vi "Advanced Buffer Configuration.vi"(0 "VISA resource name":refnum<visa-resource-name>, 1 "Enable Buffer Cache Mode (Disable)":bool, 5 "Buffer Name":string, 7 "Buffer Fill Mode (Fill_Once)":enum16{"FILL_ONCE", "FILL_WINDOW"}(ring), 9 "Buffer Fillcount":u16, 11 "error in (no error)":errorcluster) -> (4 "VISA resource name out":refnum<visa-resource-name>, 15 "error out":errorcluster)   [LabVIEW 2009, in "Keithley 2600 Series.lvlib"]
doc: "This VI allows advanced control over buffer features such as enabling cache mode, cache mode behavior and how many reading should be cached.\n\n<b>Functions and Attributes Used</b>\nbuffer.cachemode\nbuffer.fillmode\nbuffer.fillcount"
uses:
  <instrlib>/Keithley 2600 Series/Keithley 2600 Series.lvlib
  <instrlib>/Keithley 2600 Series/Private/GlobalVariables.vi
panel:
  # "(c) 2010 Keithley Instruments, Inc.  ALL RIGHTS RESERVED."
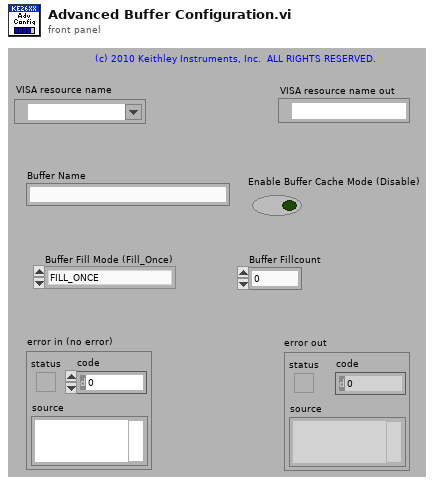
[diagram p1: front panel]
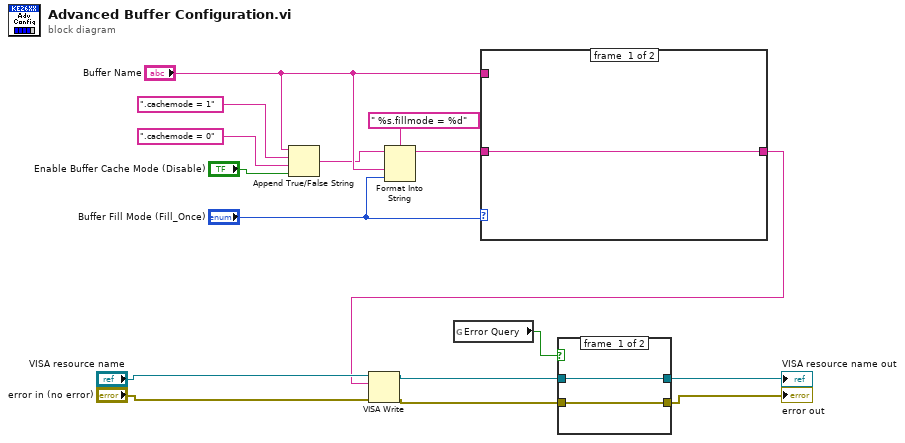
[diagram p0: block diagram]
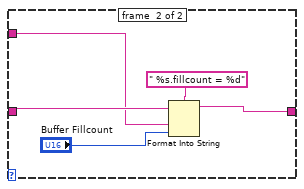
[diagram p2: hidden frame]
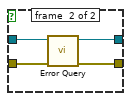
[diagram p3: hidden frame]
diagram:
  n1 = Append True/False String(1:"Enable Buffer Cache Mode (Disable)", 2:".cachemode = 0", 3:".cachemode = 1", 4:"Buffer Name") -> (0:w1:string)
  n2 = Format Into String(format string=" %s.fillmode = %d", initial string=w1, "Buffer Name", "Buffer Fill Mode (Fill_Once)") -> (resulting string=w4:string)  [unwired: 1 in, 1 out]
  n3 = global read "GlobalVariables.vi" "Error Query"() -> (w16:bool)
  n4 = case shown="\"FILL_ONCE\", Default" "Buffer Fill Mode (Fill_Once)" {
    tunnel: w4 -> [w17 w22]
    tunnel: "Buffer Name" -> [_ w21]
    tunnel: [w17 w18] -> w2
    frame #0 {
    }
    frame #1 {
      n5 = Format Into String(format string=" %s.fillcount = %d", initial string=w22, w21, "Buffer Fillcount") -> (resulting string=w18:string)  [unwired: 1 in, 1 out]
    }
  }
  n6 = VISA Write(VISA resource name="VISA resource name", write buffer=w2, error in (no error)="error in (no error)") -> (VISA resource name out=w9:refnum<visa-resource-name>, error out=w10:errorcluster)  [unwired: 1 out]
  n7 = case shown="True" w16 {
    tunnel: w9 -> [w24 w28]
    tunnel: w10 -> [w23 w27]
    tunnel: [w24 w26] -> w15
    tunnel: [w23 w25] -> w14
    frame #0 {
    }
    frame #1 {
      n8 = call <instrlib>:"Error Query.vi"("error in (no error)"=w27, "VISA resource name"=w28) -> ("error out"=w25:errorcluster, "VISA resource name out"=w26:refnum<visa-resource-name>)  [unwired: 8 out]
    }
  }
  "VISA resource name out" <- w15
  "error out" <- w14
